vi "control2contraste daq.vi"(0 "DAQ Device IN":T1={"DAQ Fs (S/s)"=10000.0, "task"="", "error"={"status"=FALSE, "code"=0, "source"=""}, "Min Value"=-10.0, "Max Value"=10.0}, 1 "Camera Device IN":T4, 2 "Image Device IN":cluster{"Image":T3, "errorImage":errorcluster}, 4 "Time Control Parameters":cluster{"# samples":u32, "tiempos (ms)":dbl}, 5 "Limites":T2, 6 "DAQ?":bool, 7 "ControlSignal":dbl[](array[numeric]), 8 "Streeam?":bool, 10 "Mostrar?":bool) -> (13 "Contraste":dbl, 14 "DAQ Device OUT":T1={"DAQ Fs (S/s)"=0.0, "task"="", "error"={"status"=FALSE, "code"=0, "source"=""}, "Min Value"=-10.0, "Max Value"=10.0}, 15 "Camara Device OUT":T4, 16 "Image Device OUT":cluster{"Image":T3, "errorImage":errorcluster}, 17 "Waveform":waveform(dbl))   [LabVIEW 2010]
uses:
  <vilib>/vision/Image Controls.llb/IMAQ Image.ctl
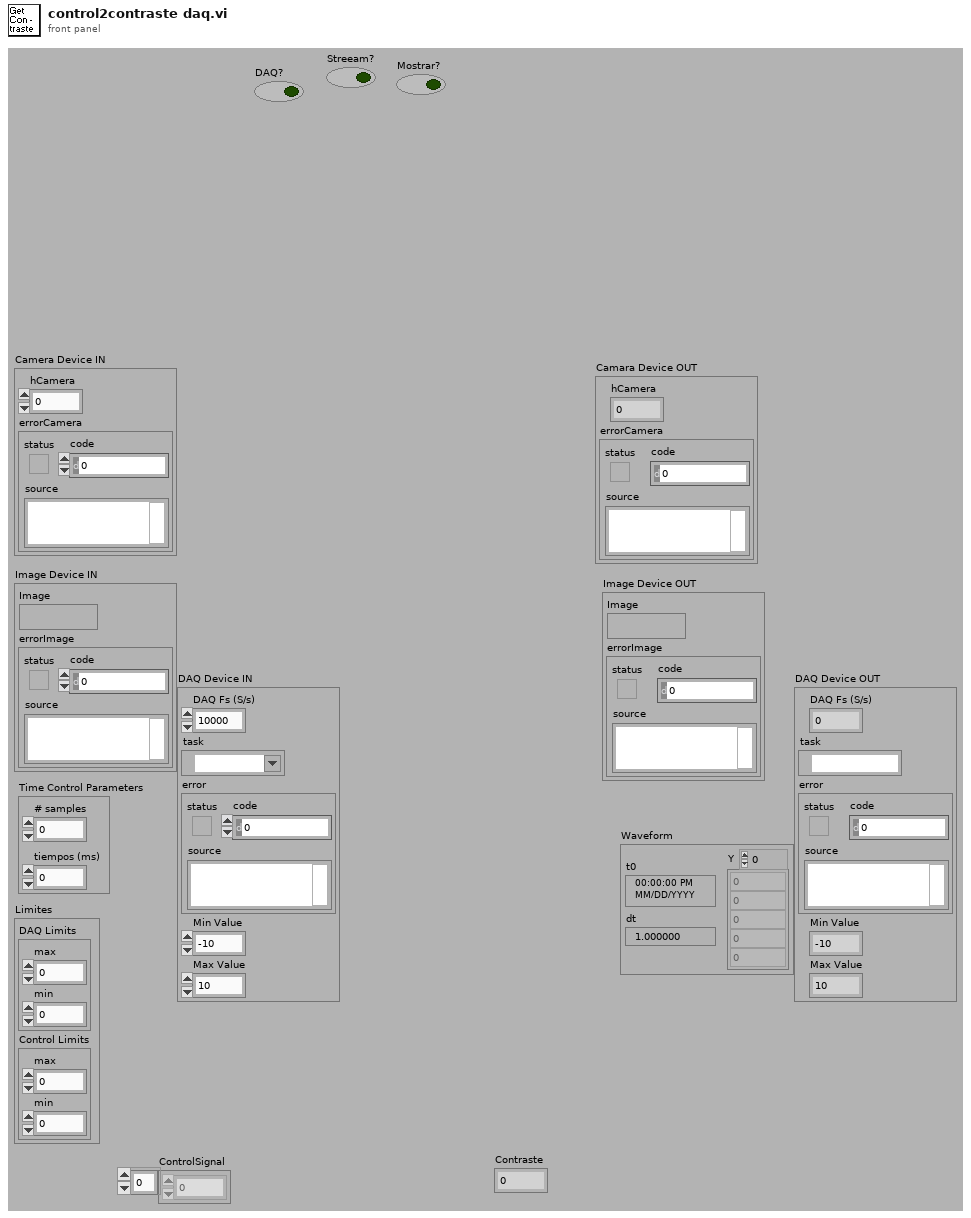
[diagram p1: front panel]
types:
  T1 = cluster{"DAQ Fs (S/s)":dbl, "task":refnum<k21>, "error":errorcluster, "Min Value":dbl, "Max Value":dbl}
  T2 = cluster{"DAQ Limits":cluster{"max":dbl, "min":dbl}, "Control Limits":cluster{"max":dbl, "min":dbl}}
  T3 = typedef "IMAQ Image.ctl" = refnum<image>
  T4 = cluster{"hCamera":u32, "errorCamera":errorcluster}
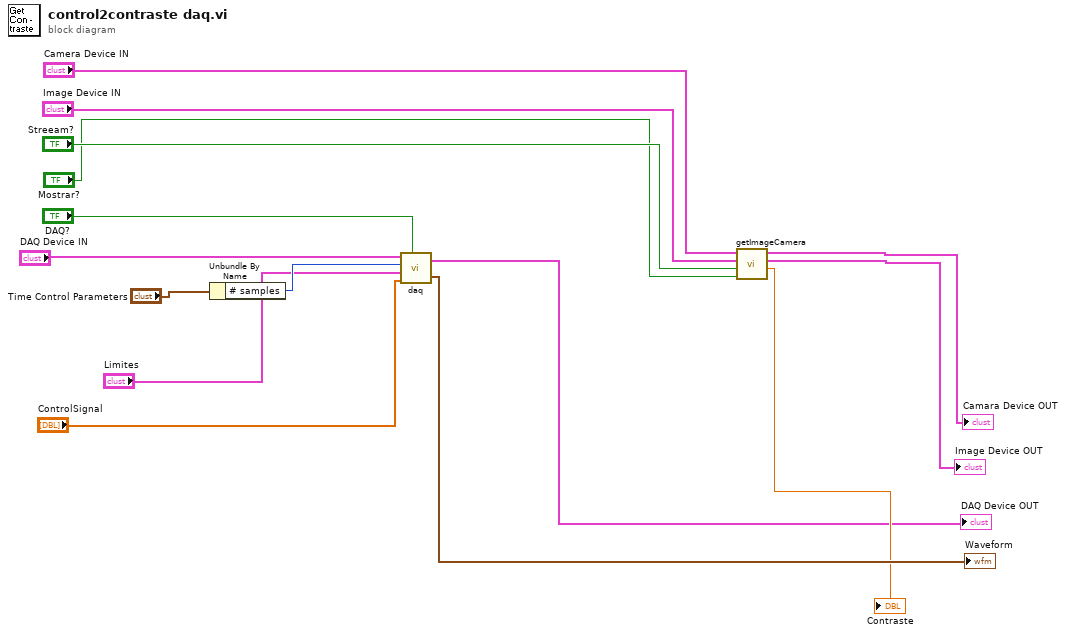
[diagram p0: block diagram]
diagram:
  n1 = Unbundle By Name("Time Control Parameters") -> ("# samples"=w4:u32)
  n2 = call "daq.vi"("DAQ Device IN"="DAQ Device IN", "#samples"=w4, "Limites"="Limites", "Control Array"="ControlSignal", "DAQ?"="DAQ?") -> ("DAQ Device OUT"=→"DAQ Device OUT":T1, "Waveform Graph"=→"Waveform":waveform(dbl))
  n3 = call "getImageCamera.vi"("Mostrar?"="Mostrar?", "Streeam?"="Streeam?", "Image Device IN"="Image Device IN", "Camera Device IN"="Camera Device IN") -> ("Contraste OUT"=→"Contraste":dbl, "Image Device OUT"=→"Image Device OUT":cluster{"Image":T3, "errorImage":errorcluster}, "Camara Device OUT"=→"Camara Device OUT":T4)  [unwired: 1 in]
